vi "Example.vi"() -> ()   [LabVIEW 2022 SP3]
uses:
  Serial_Port.xctl
  Code.xctl
panel:
  in  "Code":string(xcontrol)
  in  "Serial_Port":T2(xcontrol)
  out "Console":string
  in  "stop":bool
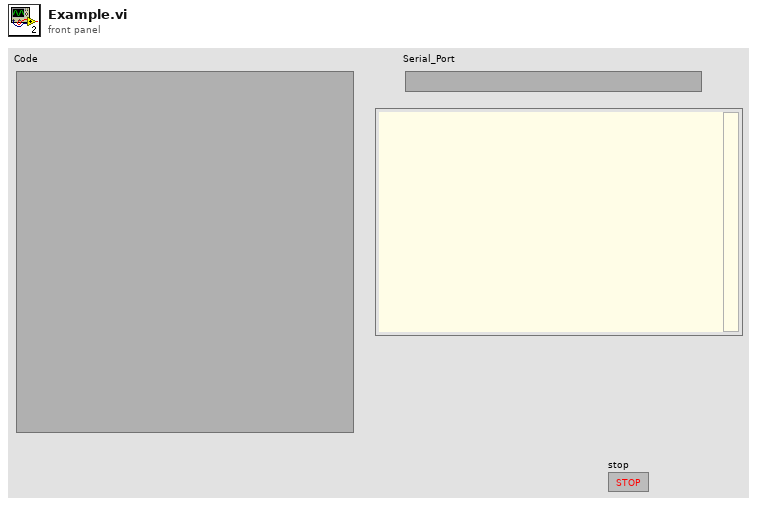
[diagram p1: front panel]
types:
  T1 = typedef "Processors.ctl" = enum16{"SPIKE", "Pi", "Pi_ssh", "OpenMV", "Dunio"}
  T2 = cluster{"session":refnum<k35>, "PyPath":path, "Processor":T1, "Port":string, "version":string}
  T3 = typedef "PythonCtrl.ctl" = cluster{"session":refnum<k35>, "PyPath":path, "Processor":T1, "Port":string, "version":string}
  T4 = enum8{"Enabled", "Disabled", "Disabled and Grayed Out"}
  T5 = typedef "eventvkey.ctl" = enum16{"ASCII", "Enter", "Return", "Shift", "Ctrl", "Alt", "Cmd", "Opt", "Caps", "NumLock", "Clear", "Break", "Up", "Down", "Left", "Right", "Insert", "Delete", "Home", "End", "PageUp", "PageDown", "Escape", "Help", "Pause", "ScrollLock", "F1", "F2", "F3", "F4", "F5", "F6", "F7", "F8", "F9", "F10", "F11", "F12", "F13", "F14", "F15", "F16", "F17", "F18", "F19", "F20", "F21", "F22", "F23", "F24", "Play", "VolumeUp", "VolumeDown", "Mute", "Two Byte Char"}
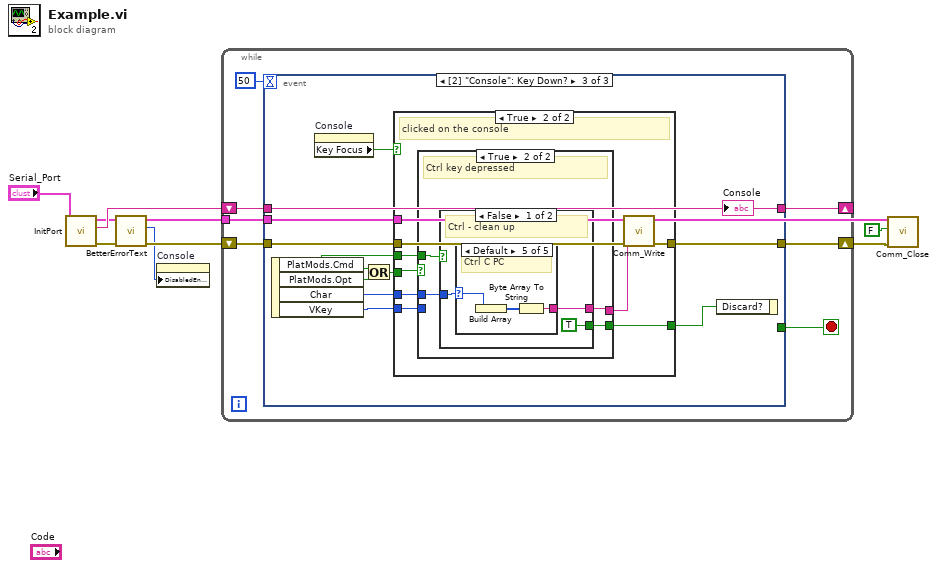
[diagram p0: block diagram]
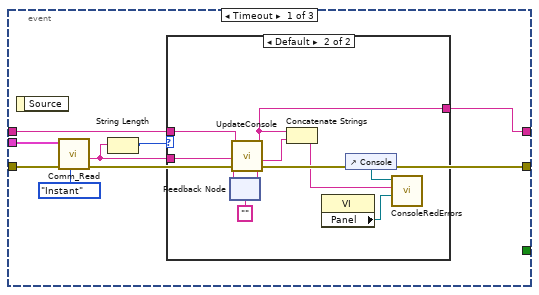
[diagram p2: hidden frame]
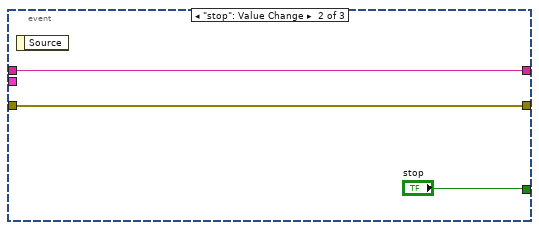
[diagram p4: hidden frame]
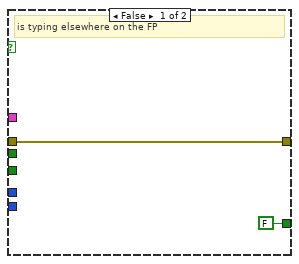
[diagram p5: hidden frame]
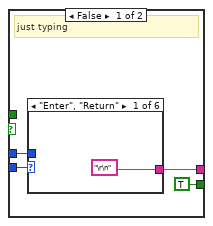
[diagram p6: hidden frame]
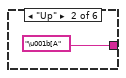
[diagram p7: hidden frame]
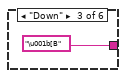
[diagram p8: hidden frame]
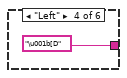
[diagram p9: hidden frame]
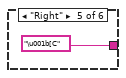
[diagram p10: hidden frame]
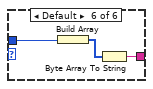
[diagram p11: hidden frame]
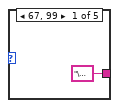
[diagram p12: hidden frame]
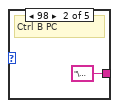
[diagram p13: hidden frame]
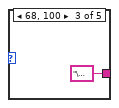
[diagram p14: hidden frame]
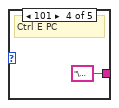
[diagram p15: hidden frame]
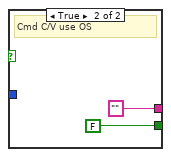
[diagram p16: hidden frame]
diagram:
  n1 = call "InitPort.vi"("Python"="Serial_Port") -> ("error out"=w4:errorcluster, "Console"=w5:string, "Python out"=w2:T3)  [unwired: 8 in]
  n2 = call "BetterErrorText.vi"("error in (no error)"=w4, "Python"=w2) -> ("Disabled"=w3:T4, "Python out"=w7:T3)  [unwired: 8 in]
  n3 = property on="Console" class="Str"("DisabledEnum"=w3) -> ()  [unwired: 2 in, 2 out]
  n4 = while {
    tunnel: w7 -> [w14]
    shift-right: [w12] -> w8
    shift-left: w4 -> [w15]
    shift-right: [w9] -> _
    shift-left: w5 -> [w13]
    stop <- w10 stop-if-true
    n5 = event shown="[2] \"Console\": Key Down?" {
      selector: _ -> [_ _ _]
      dyn-events: _ -> [_ _ _]
      timeout: u32 50 ("milliseconds to wait") -> [_ _ _]
      tunnel: w15 -> [w23 w36 w48]
      tunnel: w14 -> [w21 _ w47]
      tunnel: w13 -> [w20 w35 w39]
      tunnel: [w19 w36 w46] -> w12
      tunnel: [_ "stop" _] -> w10
      tunnel: [w18 w35 w39] -> w9
      event Timeout {
        n6 = event-data() -> ()  [unwired: 1 in, 1 out]
        n7 = call "Comm_Read.vi"("Task"=enum16{"Instant", "All", "AllFast", "Params"}."Instant", "error in (no error)"=w23, "Python"=w21) -> ("error out"=w19:errorcluster, "Text read"=w17:string)  [unwired: 7 in]
        n8 = String Length(string=w17) -> (length=w16:i32)
        n9 = case shown="Default" w16 {
          tunnel: w17 -> [_ w31]
          tunnel: w20 -> [w24 w30]
          tunnel: [w24 w25] -> w18
          frame 0 {
          }
          frame Default {
            n10 = feedback #1("" ("Left over raw")) -> (w34:string)
            n11 = call "UpdateConsole.vi"("from last time raw"=w34, "New Text"=w31, "Console"=w30) -> ("Left over raw"=w32:string, "left over fixed"=w28:string, "Console Out"=w25:string)  [unwired: 4 in, 2 out]
            n12 = feedback-in #1(w32) -> ()
            n13 = Concatenate Strings(w25, w28) -> (w26:string)
            n14 = property class="VI"() -> ("Panel"=w27:refnum<vi>)  [unwired: 2 in, 2 out]
            n15 = control-ref of="Console"() -> (w29:refnum<vi>)
            n16 = call "ConsoleRedErrors.vi"("Front Panel"=w27, "Console in"=w26, "String in"=w29) -> ()  [unwired: 7 in, 2 out]
          }
        }
      }
      event "stop": Value Change {
        n17 = event-data() -> ()  [unwired: 1 in, 1 out]
      }
      event "Console": Key Down? {
        n18 = event-data() -> ("PlatMods.Cmd"=w40:bool, "PlatMods.Opt"=w43:bool, "Char"=w44:i16, "VKey"=w45:T5)  [unwired: 1 in]
        n19 = property on="Console" class="Str"() -> ("Key Focus"=w38:bool)  [unwired: 2 in, 2 out]
        n20 = Or(x=w40, y=w43) -> (x .or. y?=w42:bool)
        n21 = case shown="True" w38 {
          tunnel: w48 -> [w50 w58]
          tunnel: w47 -> [_ w57]
          tunnel: [w50 w56] -> w46
          tunnel: w45 -> [_ w55]
          tunnel: w44 -> [_ w54]
          tunnel: w42 -> [_ w53]
          tunnel: [FALSE ("Discard?") w52] -> w41
          tunnel: w40 -> [_ w51]
          frame False {
            # "is typing elsewhere on the FP"
          }
          frame True {
            # "clicked on the console"
            n22 = case shown="True" w53 {
              tunnel: [w63 w74] -> w59
              tunnel: w55 -> [w62 _]
              tunnel: w54 -> [w61 w75]
              tunnel: [TRUE ("Discard?") w73] -> w52
              tunnel: w51 -> [_ w72]
              frame False {
                # "just typing"
                n23 = case shown="\"Enter\", \"Return\"" w62 {
                  tunnel: w61 -> [_ _ _ _ _ w71]
                  tunnel: ["\r\n" ("replace string (\"\")") "\u001b[A" ("replace string (\"\")") "\u001b[B" ("replace string (\"\")") "\u001b[D" ("replace string (\"\")") "\u001b[C" ("replace string (\"\")") w69] -> w63
                  frame "Enter", "Return" {
                  }
                  frame "Up" {
                  }
                  frame "Down" {
                  }
                  frame "Left" {
                  }
                  frame "Right" {
                  }
                  frame Default {
                    n24 = Build Array(w71) -> (w70:i16[])
                    n25 = Byte Array To String(unsigned byte array=w70) -> (string=w69:string)
                  }
                }
              }
              frame True {
                # "Ctrl key depressed"
                n26 = case shown="False" w72 {
                  tunnel: [w78 "" ("string")] -> w74
                  tunnel: w75 -> [w77 _]
                  tunnel: [TRUE ("Discard?") FALSE ("Discard?")] -> w73
                  frame False {
                    # "Ctrl - clean up"
                    n27 = case shown="Default" w77 {
                      selector: w77 -> [_ _ _ _ w83]
                      tunnel: ["\u0003" ("string") "\u0002" ("string") "\u0004" ("string") "\u0005" ("string") w84] -> w78
                      frame 67, 99 {
                      }
                      frame 98 {
                        # "Ctrl B PC"
                      }
                      frame 68, 100 {
                      }
                      frame 101 {
                        # "Ctrl E PC"
                      }
                      frame Default {
                        # "Ctrl C PC"
                        n28 = Build Array(w83) -> (w85:i16[])
                        n29 = Byte Array To String(unsigned byte array=w85) -> (string=w84:string)
                      }
                    }
                  }
                  frame True {
                    # "Cmd C/V use OS"
                  }
                }
              }
            }
            n30 = call "Comm_Write.vi"("error in (no error)"=w58, "Text to write"=w59, "Python"=w57) -> ("error out"=w56:errorcluster)  [unwired: 7 in, 1 out]
          }
        }
        n31 = event-data("Discard?"=w41) -> ()  [unwired: 1 in, 1 out]
        "Console" <- w39
      }
    }
  }
  n32 = call "Comm_Close.vi"("error in (no error)"=w8, "Show Err?"=FALSE, "Python in"=w7) -> ()  [unwired: 7 in, 2 out]
